vi "ConfigureInstrument.vi"(8 "error in (no error)":errorcluster, 11 "PalmSens in":refnum<class "PalmSens.lvclass">) -> (0 "error out":errorcluster, 2 "PSLabView Instance":refnum<k24>, 3 "PalmSens out":refnum<class "PalmSens.lvclass">)   [LabVIEW 2025, in "PalmSens.lvclass"]
uses:
  PalmSens.lvclass
  E:/PSCode/PalmSens_SDK/labview/PalmSens/Libraries/PalmSens.Core.Simplified.LabVIEW.dll
  Libraries/PalmSens.Core.Simplified.LabVIEW.dll
  PalmSens.lvclass/PalmSens.ctl
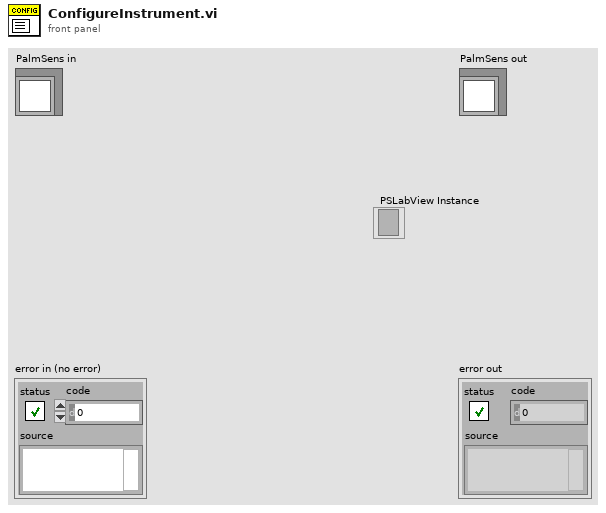
[diagram p1: front panel]
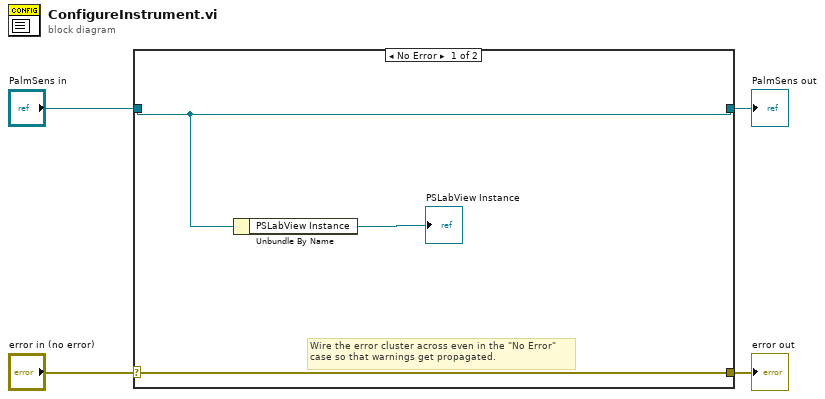
[diagram p0: block diagram]
diagram:
  n1 = case shown="No Error" "error in (no error)" {
    selector: "error in (no error)" -> [w7 w9]
    tunnel: [w7 w9] -> w3
    tunnel: [w6 w8] -> w1
    tunnel: "PalmSens in" -> [w6 w8]
    frame No Error {
      # "Wire the error cluster across even in the \"No Error\"\ncase so that warnings get propagated."
      n2 = Unbundle By Name(w6) -> ("PSLabView Instance"=→"PSLabView Instance":refnum<k24>)
    }
    frame Error {
    }
  }
  "error out" <- w3
  "PalmSens out" <- w1
